vi "DAQ@CompareAvgInRange__Parameter.vi"(1 "ParamterIn":string) -> (0 "ParamterOut":string)   [LabVIEW 2020]
panel:
  in  "End":string(combo)
  in  "Start":string(combo)
  in  "Min":string(combo)
  in  "Max":string(combo)
  in  "WaveFormName":string(combo)
  in  "Confirm":bool
  # "~"
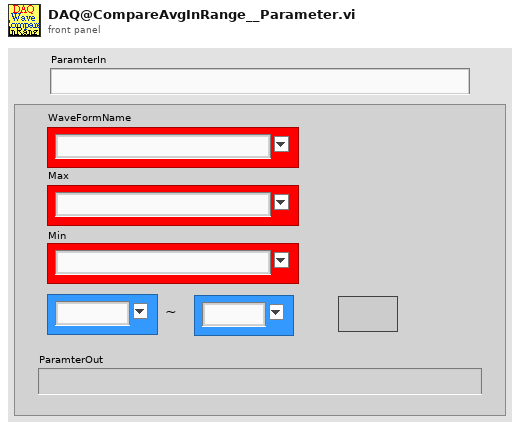
[diagram p1: front panel]
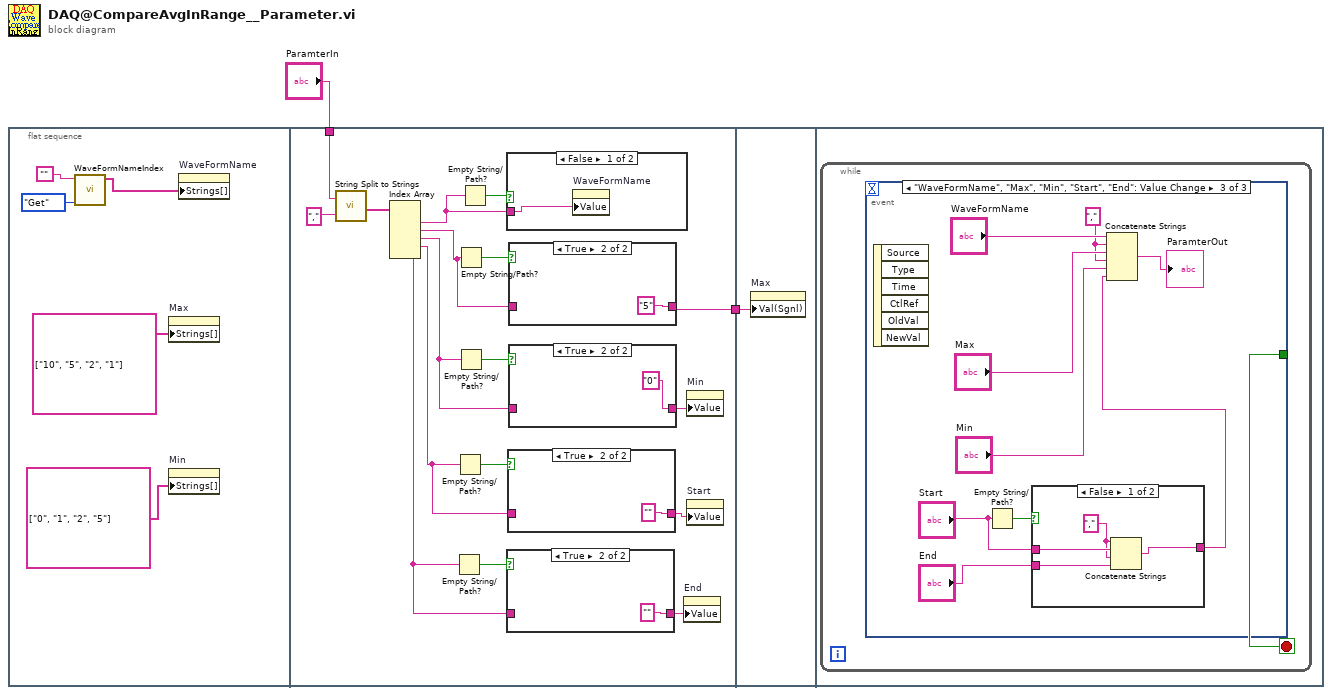
[diagram p0: block diagram]
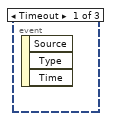
[diagram p7: hidden frame]
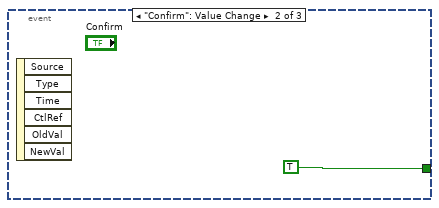
[diagram p8: hidden frame]
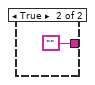
[diagram p9: hidden frame]
diagram:
  n1 = flat-sequence {
    tunnel: "ParamterIn" -> [w22]
    tunnel: [w8] -> w1
    tunnel: w1 -> [w34]
    frame #0 {
      n2 = call "WaveFormNameIndex.vi"("OP"=enum16{"Get", "Update", "Init", "GetSPS"}."Get", "WaveFormName"="") -> ("WaveFormNameList"=w5:string[])  [unwired: 6 in, 3 out]
      n3 = property on="Max" class="CmbBox"("Strings[]"=string[] ["10", "5", "2", "1"] ("Strings []")) -> ()  [unwired: 2 in, 2 out]
      n4 = property on="Min" class="CmbBox"("Strings[]"=string[] ["0", "1", "2", "5"] ("Strings []")) -> ()  [unwired: 2 in, 2 out]
      n5 = property on="WaveFormName" class="CmbBox"("Strings[]"=w5) -> ()  [unwired: 2 in, 2 out]
    }
    frame #1 {
      n6 = call "String Split to Strings.vi"("search string/char (-)"=",", "String"=w22) -> ("Array"=w21:string[])
      n7 = Index Array(array=w21) -> (element #1=w20:string, element #2=w18:string, element #3=w16:string, element #4=w13:string, element #5=w10:string)  [unwired: 5 in]
      n8 = Empty String/Path?(string/path=w10) -> (empty?=w11:bool)
      n9 = Empty String/Path?(string/path=w13) -> (empty?=w14:bool)
      n10 = Empty String/Path?(string/path=w18) -> (empty?=w19:bool)
      n11 = Empty String/Path?(string/path=w16) -> (empty?=w17:bool)
      n12 = Empty String/Path?(string/path=w20) -> (empty?=w24:bool)
      n13 = case shown="False" w24 {
        tunnel: w20 -> [w33 _]
        frame False {
          n14 = property on="WaveFormName" class="CmbBox"("Value"=w33) -> ()  [unwired: 2 in, 2 out]
        }
        frame True {
        }
      }
      n15 = case shown="True" w11 {
        tunnel: w10 -> [w25 _]
        tunnel: [w25 ""] -> w9
        frame False {
        }
        frame True {
        }
      }
      n16 = case shown="True" w14 {
        tunnel: w13 -> [w27 _]
        tunnel: [w27 ""] -> w12
        frame False {
        }
        frame True {
        }
      }
      n17 = case shown="True" w19 {
        tunnel: w18 -> [w31 _]
        tunnel: [w31 "5"] -> w8
        frame False {
        }
        frame True {
        }
      }
      n18 = case shown="True" w17 {
        tunnel: w16 -> [w29 _]
        tunnel: [w29 "0"] -> w15
        frame False {
        }
        frame True {
        }
      }
      n19 = property on="End" class="CmbBox"("Value"=w9) -> ()  [unwired: 2 in, 2 out]
      n20 = property on="Min" class="CmbBox"("Value"=w15) -> ()  [unwired: 2 in, 2 out]
      n21 = property on="Start" class="CmbBox"("Value"=w12) -> ()  [unwired: 2 in, 2 out]
    }
    frame #2 {
      n22 = property on="Max" class="CmbBox"("Val(Sgnl)"=w34) -> ()  [unwired: 2 in, 2 out]
    }
    frame #3 {
      n23 = while {
        stop <- w35 stop-if-true
        n24 = event shown="[2] \"WaveFormName\", \"Max\", \"Min\", \"Start\", \"End\": Value Change" {
          selector: _ -> [_ _ _]
          dyn-events: _ -> [_ _ _]
          timeout: _ -> [_ _ _]
          tunnel: [_ TRUE _] -> w35
          event Timeout {
            n25 = event-data() -> ()  [unwired: 1 in, 3 out]
          }
          event "Confirm": Value Change {
            n26 = event-data() -> ()  [unwired: 1 in, 6 out]
          }
          event "WaveFormName", "Max", "Min", "Start", "End": Value Change {
            w41 = ","
            n27 = event-data() -> ()  [unwired: 1 in, 6 out]
            n28 = Empty String/Path?(string/path="Start") -> (empty?=w40:bool)
            n29 = case shown="False" w40 {
              tunnel: [w49 ""] -> w39
              tunnel: "Start" -> [w48 _]
              tunnel: "End" -> [w47 _]
              frame False {
                w46 = ","
                n30 = Concatenate Strings(w46, w48, w46, w47) -> (w49:string)
              }
              frame True {
              }
            }
            n31 = Concatenate Strings("WaveFormName", w41, "Max", w41, "Min", w39) -> (→"ParamterOut":string)
          }
        }
      }
    }
  }
